vi "subConvertQAMM-AryEnumtoNum.vi"(1 "QAM M-ary":enum16{"4", "8", "16", "32", "64", "128", "256"}(ring)) -> (0 "M-QAM":i32)   [LabVIEW 2015]
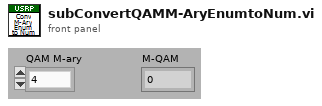
[diagram p1: front panel]
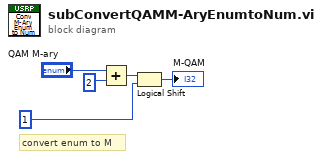
[diagram p0: block diagram]
diagram:
  # "convert enum to M"
  n1 = Add(x="QAM M-ary", y=2) -> (x+y=w2:i32)
  n2 = Logical Shift(y=w2, x=1) -> (x << y=→"M-QAM":i32)
